vi "remoteControlShooter.vi"() -> ()   [LabVIEW 2019]
uses:
  <vilib>/ReMiSYS/ReMiSYS_myRIO-mini/SubVI/gamepadF710/F710.ctl
  <vilib>/ReMiSYS/ReMiSYS_myRIO-mini/SubVI/gamepadF710/stick.ctl
  <vilib>/ReMiSYS/ReMiSYS_myRIO-mini/SubVI/gamepadF710/gamepadF710.lvclass
  <vilib>/Platform/TimedLoop/XDataNode/timing_clust.ctl
  <vilib>/Platform/TimedLoop/XDataNode/nitl_modes.ctl
  <vilib>/Platform/TimedLoop/XDataNode/wakeup.ctl
  <vilib>/ReMiSYS/ReMiSYS_myRIO-mini/SubVI/SYS/servoPort.ctl
  <vilib>/myRIO/Common/Instrument Driver Framework/myRIO v1.0/UART/vis/myRIO v1.0 Close UART.vi
  <vilib>/myRIO/Common/Instrument Driver Framework/Utilities/vis/FPGA Ref Manager.vi
  <vilib>/myRIO/Common/Instrument Driver Framework/myRIO v1.0/myRIO v1.0 Reset FPGA.vi
  <vilib>/myRIO/Common/Instrument Driver Framework/myRIO v1.0/IRQ/vis/myRIO v1.0 IRQ Info FGV.vi
  <vilib>/myRIO/Common/Instrument Driver Framework/myRIO v1.0/IRQ/vis/myRIO v1.0 Timer IRQ Info FGV.vi
  <vilib>/myRIO/Common/Instrument Driver Framework/myRIO v1.0/IRQ/vis/myRIO v1.0 ISR Agent.vi
  <vilib>/myRIO/Instrument Drivers/Utilities/vis/Reset Index.vi
  <vilib>/myRIO/Common/Instrument Driver Framework/myRIO v1.0/Resource Manager/vis/myRIO v1.0 Block Write Resource Manager.vi
  <vilib>/Platform/TimedLoop/XDataNode/XDataNode.xnode
  <vilib>/Platform/TimedLoop/XDataNode/XDNodeRunTimeDep.lvlib
  <vilib>/myRIO/Instrument Drivers/Utilities/Utilities.lvlib
  <vilib>/vision/Image Controls.llb/IMAQ Image.ctl
panel:
  out "Image Out":T1(plugin-control)
  out "sorted circles by center x then y":T2(array[cluster])
  out "i":i32
  in  "Circle Descriptor (Shape Detection 1)":cluster{"Min Radius":dbl, "Max Radius":dbl}={"Min Radius"=30.0, "Max Radius"=300.0}
  in  "read image\nalgorithm":bool=TRUE
  out "error out":errorcluster
  out "Position.x":sgl
  out "Position.y":sgl
  out "F710 button info.LogiB":bool
  in  "speed 1~10":dbl=10.0
  out "shooterPitch":dbl
  out "ClipCtrl":bool[](array[boolean])
  out "Speed Array":dbl[](array[numeric])
  in  "stop Control?":bool
  out "F710":T3
  out "ENC [L, R, B] (deg)":dbl[](array[numeric])
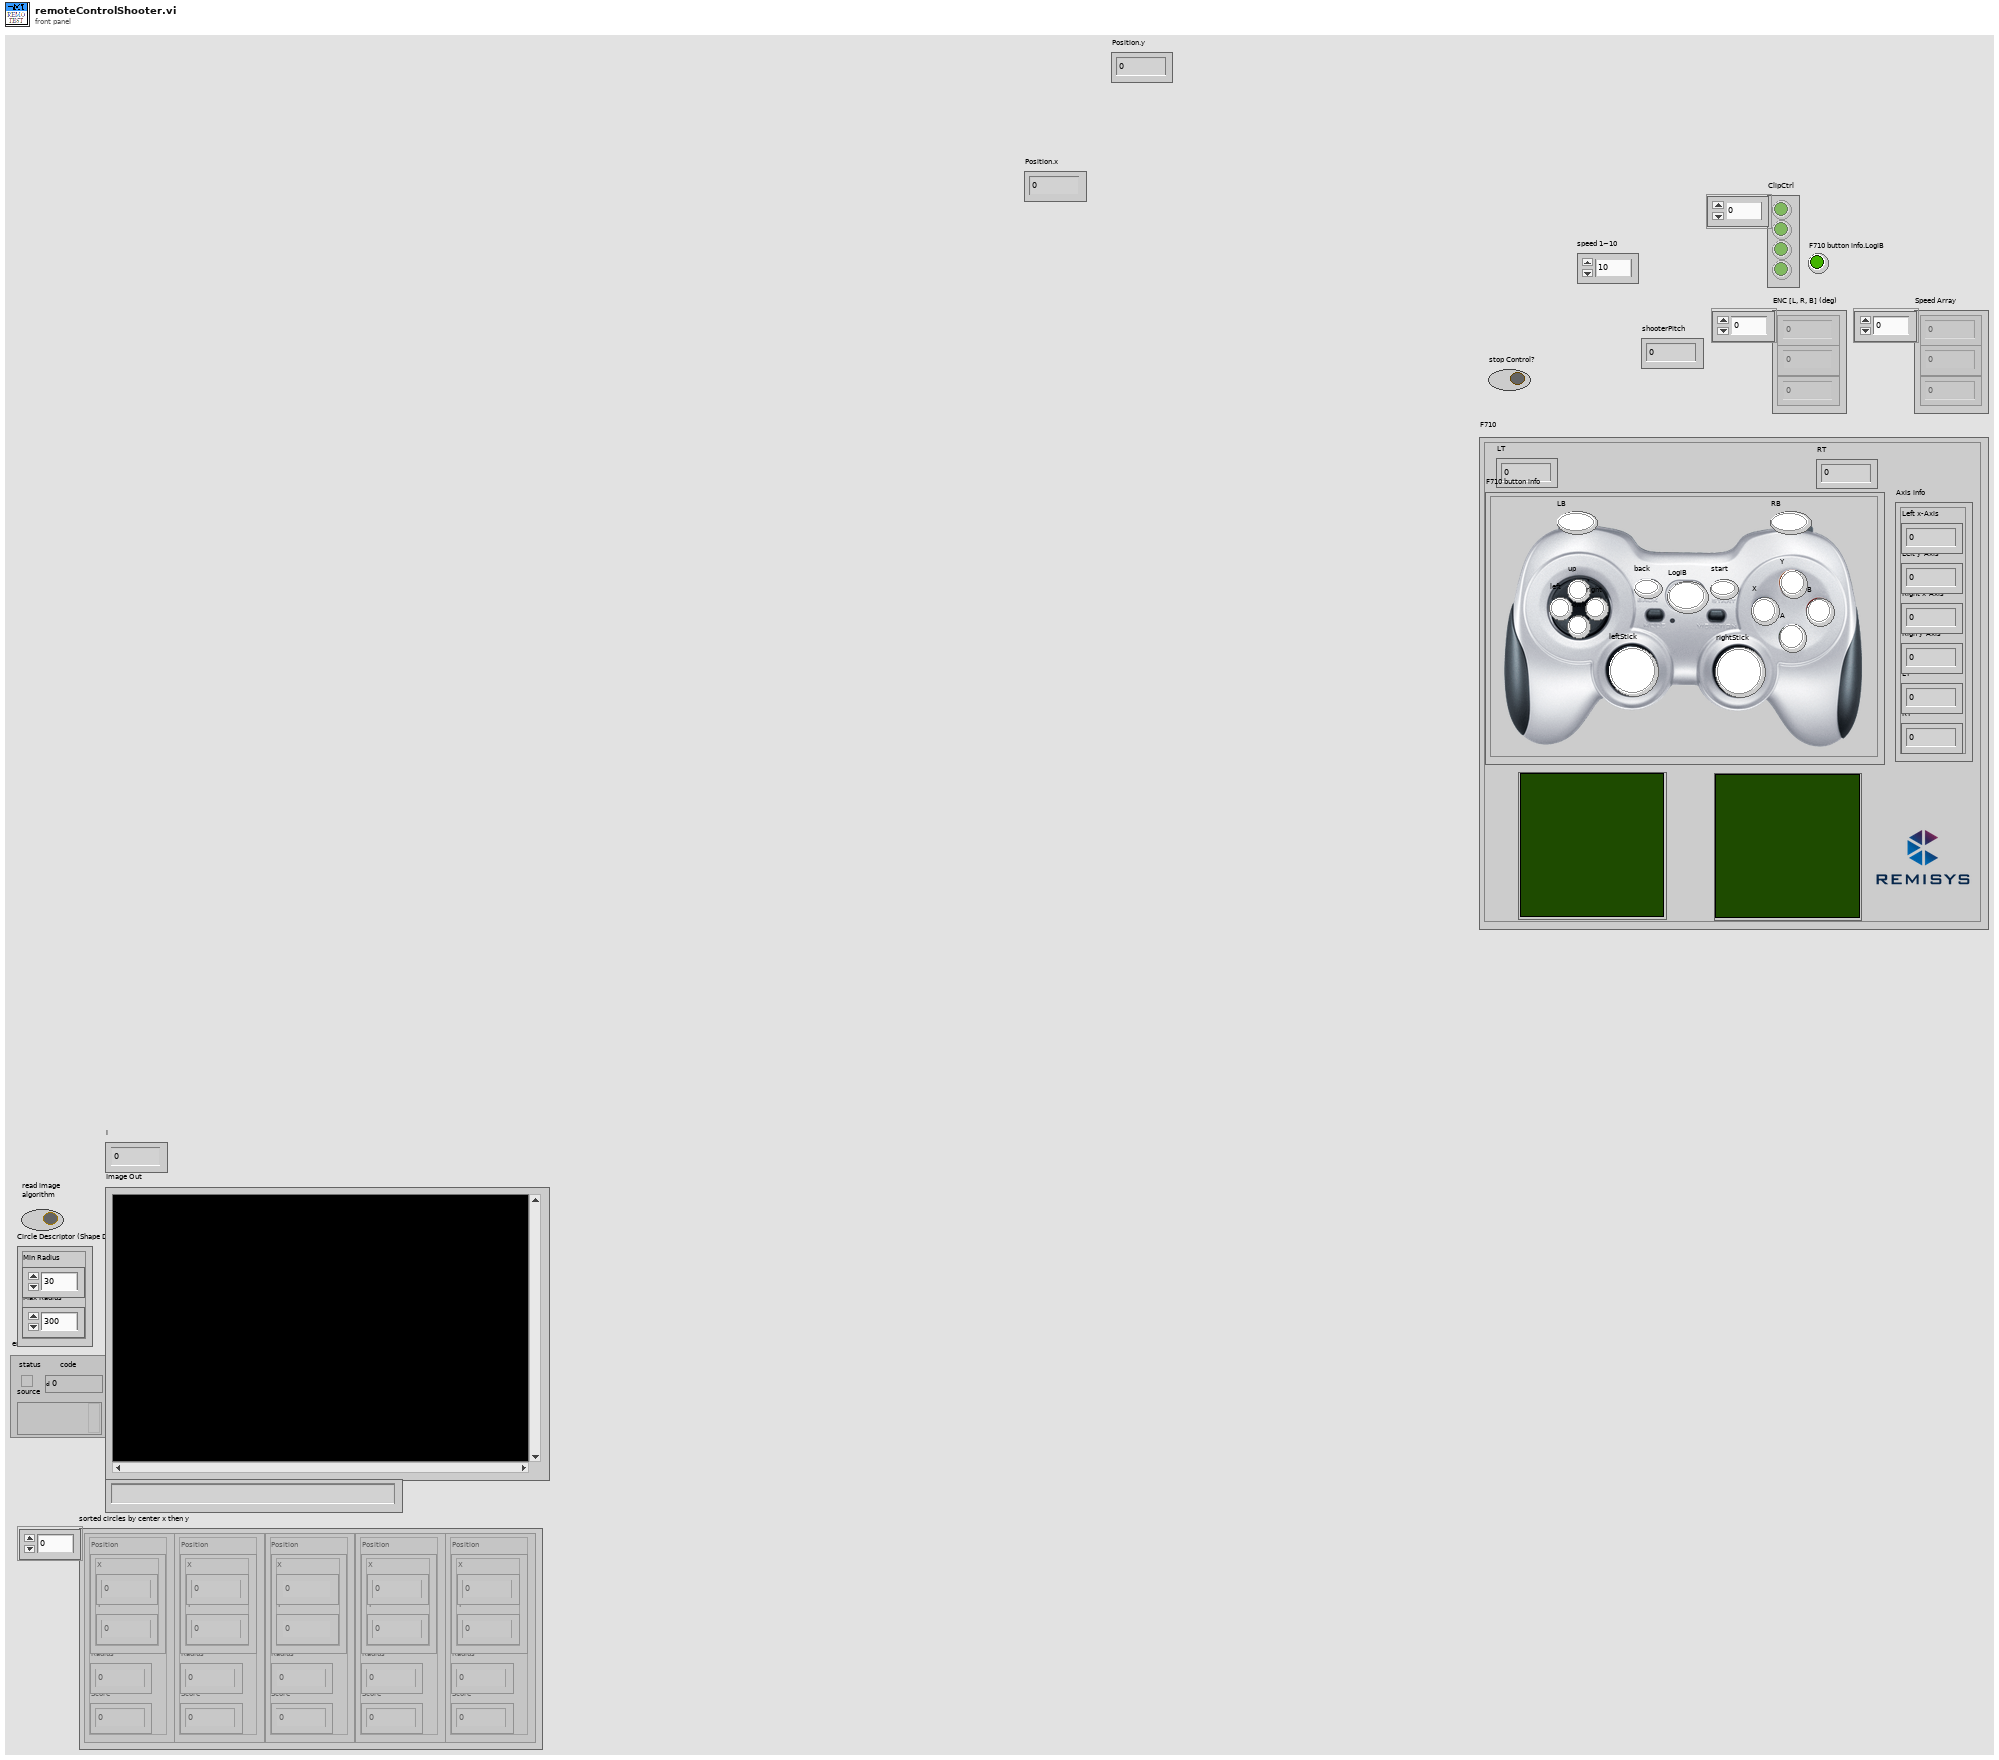
[diagram p1: front panel]
types:
  T1 = typedef "IMAQ Image.ctl" = refnum<image>
  T2 = cluster{"Position":cluster{"X":u16, "Y":u16}, "Radius":u16, "Score":u16}[]
  T3 = typedef "F710.ctl" = cluster{"RT":u8, "LT":u8, "RightStick":T4, "LeftStick":T4, "Axis info":cluster{"Left x-Axis":i8, "Left y-Axis":i8, "Right x-Axis":i8, "Righ y-Axis":i8, "LT":u8, "RT":u8}, "F710 button info":cluster{"RB":bool, "LB":bool, "rightStick":bool, "leftStick":bool, "start":bool, "back":bool, "right":bool, "left":bool, "down":bool, "up":bool, "Y":bool, "X":bool, "B":bool, "A":bool, "LogiB":bool}}
  T4 = typedef "stick.ctl" = cluster{"X":dbl, "Y":dbl}[]
  T5 = cluster{"Position":cluster{"X":sgl, "Y":sgl}, "Radius":dbl, "Score":dbl}[]
  T6 = typedef "Image Type" = u32
  T7 = cluster{"Position":cluster{"X":u16, "Y":u16}, "Radius":u16, "Score":u16}
  T8 = typedef "servoPort.ctl" = enum16{"S1", "S2", "S3", "S4", "S5", "S6", "S7", "S8", "S9"}
  T9 = typedef "XDNodeRunTimeDep.lvlib/timing_clust.ctl" = cluster{"Expected End [f-1]":u64, "Actual End [f-1]":u64, "Finished Late? [f-1]":bool, "Expected End [i-1]":u64, "Actual End [i-1]":u64, "Finished Late? [i-1]":bool, "Expected Start [i]":u64, "Actual Start [i]":u64, "Expected Start [f]":u64, "Actual Start [f]":u64, "Source Name":string, "Structure Name":string, "Period":i64, "Deadline":i64, "Offset":i64, "Start":i64, "Priority":i32, "Timeout":i32, "Mode":T10, "Wakeup Reason":T11, "Error":errorcluster, "Source Type":string, "Secondary Source Type":string, "Global End Time":u64, "Global Start Time":u64, "Frame Duration":u64, "Iteration Duration":u64, "Assigned CPU":i32, "I/O Scan Engine Mode":u32}
  T10 = typedef "XDNodeRunTimeDep.lvlib/nitl_modes.ctl" = enum32{"No Change", "Process missed periods, maintain original phase", "Discard missed periods, maintain original phase", "Process missed periods, ignore original phase", "Discard missed periods, ignore original phase"}
  T11 = typedef "XDNodeRunTimeDep.lvlib/wakeup.ctl" = enum32{"Normal", "Aborted", "Asynchronous wakeup", "Timing source error", "Timed loop error", "Timeout"}
  T12 = typedef "miniRef.ctl" = cluster{"Custom FPGA Reference":refnum<k20>, "error out":errorcluster}
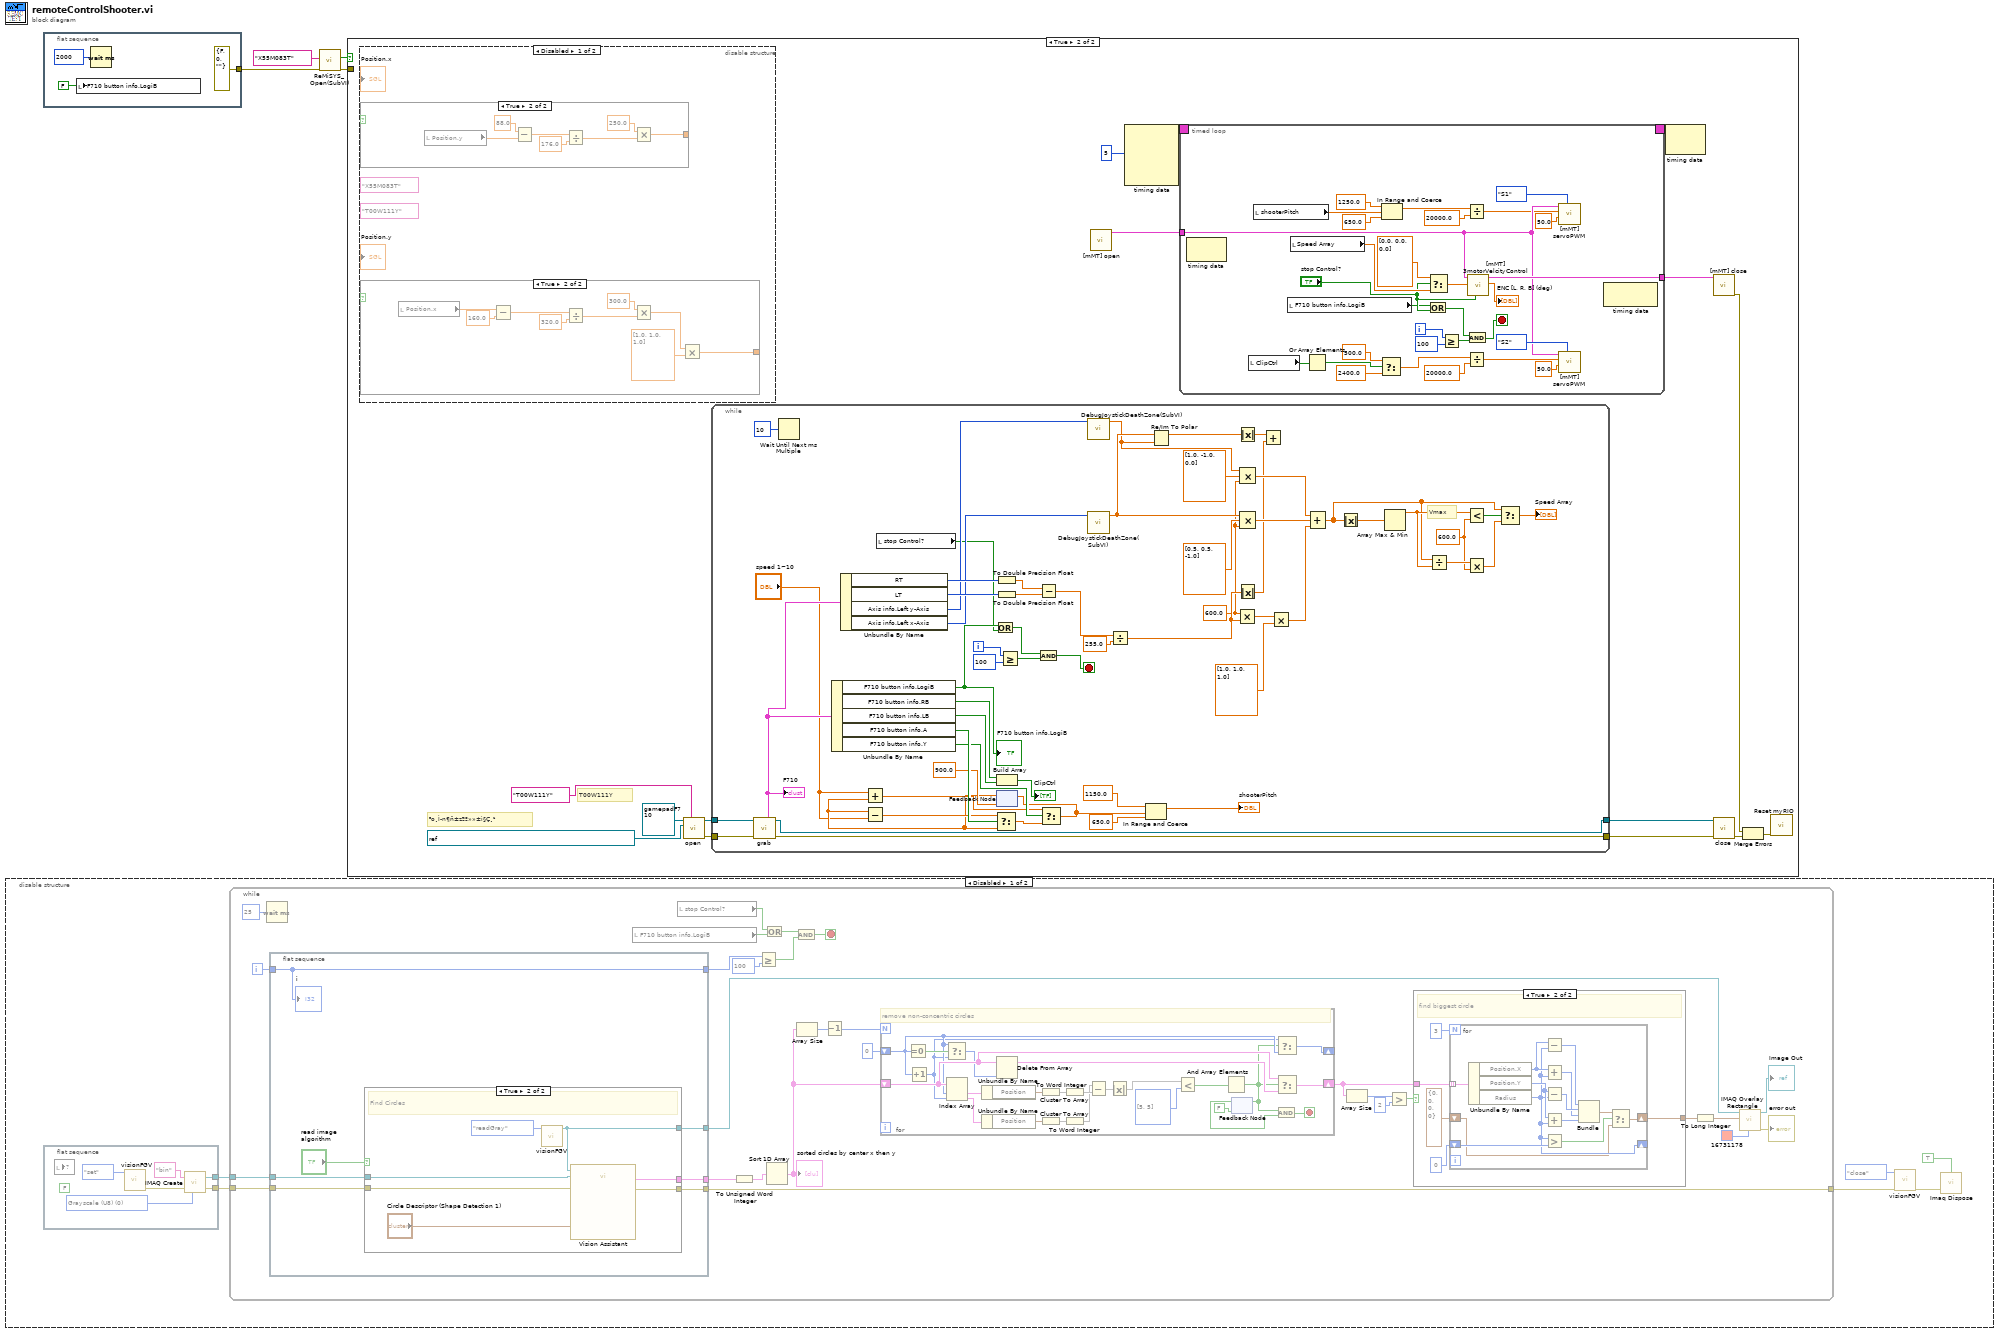
[diagram p0: block diagram]
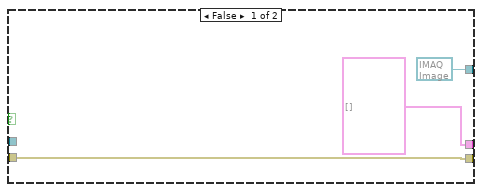
[diagram p2: hidden frame]
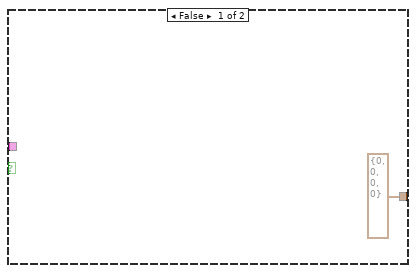
[diagram p3: hidden frame]
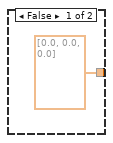
[diagram p6: hidden frame]
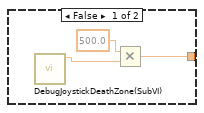
[diagram p7: hidden frame]
diagram:
  n1 = disable-structure shown="Disabled" {
    frame Disabled {
      n2 = flat-sequence {
        tunnel: [w15] -> w10
        tunnel: [w13] -> w7
        frame #0 {
          (unwired) FALSE ("stop Control?")
          w14 = T6 0 items=["Grayscale (U8)", "Grayscale (I16)", "Grayscale (SGL)", "Complex (CSG)", "RGB (U32)", "HSL (U32)", "RGB (U64)", "Grayscale (U16)"] ("Image Type")
          n3 = local read item#-1() -> ()  [unwired: 1 in]
          n4 = call "visionFGV.vi"("Function"=enum16{"set", "readColor", "close", "readGray"}."set") -> ("error out"=w11:errorcluster)  [unwired: 9 in, 1 out]
          n5 = call "IMAQ Create"("Image Name"="bin", "Image Type"=w14, "error in (no error)"=w11) -> ("New Image"=w15:T1, "error out"=w13:errorcluster)  [unwired: 2 in]
        }
      }
      n6 = while {
        tunnel: [w35] -> w6
        tunnel: w10 -> [w44]
        tunnel: w7 -> [w29]
        i -> [w40]
        stop <- w18 stop-if-true
        n7 = Wait (ms)(milliseconds to wait=u32 25) -> ()  [unwired: 1 out]
        n8 = flat-sequence {
          tunnel: [w50] -> w35
          tunnel: [w48] -> w32
          tunnel: [w46] -> w28
          tunnel: w44 -> [w51]
          tunnel: w40 -> [w45]
          tunnel: w29 -> [w47]
          tunnel: [w45] -> w17
          frame #0 {
            n9 = case shown="True" "read image\nalgorithm" {
              tunnel: [w53 w59] -> w50
              tunnel: w51 -> [_ w61]
              tunnel: [T5 [] ("Circles (Shape Detection 1)") w60] -> w48
              tunnel: w47 -> [w53 w57]
              tunnel: [T1 refnum ("Image Out fgv") w55] -> w46
              frame False {
              }
              frame True {
                # "Find Circles"
                n10 = call "visionFGV.vi"("Function"=enum16{"set", "readColor", "close", "readGray"}."readGray") -> ("Image Out fgv"=w55:T1)  [unwired: 9 in, 1 out]
                n11 = call "Vision Assistant"("Image In"=w55, "Image Dst"=w61, "Circle Descriptor (Shape Detection 1)"="Circle Descriptor (Shape Detection 1)", "error in"=w57) -> ("Circles (Shape Detection 1)"=w60:T5, "error out"=w59:errorcluster)  [unwired: 21 in, 1 out]
              }
            }
            "i" <- w45
          }
        }
        n12 = local read "F710 button info.LogiB"() -> (w21:bool)
        n13 = local read "stop Control?"() -> (w22:bool)
        n14 = To Unsigned Word Integer(number=w32) -> (unsigned 16bit integer=w39:T2)
        n15 = Greater Or Equal?(x=w17, y=100) -> (x >= y?=w19:bool)
        n16 = Or(x=w22, y=w21) -> (x .or. y?=w20:bool)
        n17 = Sort 1D Array(array=w39) -> (sorted array=w36:T2)
        "sorted circles by center x then y" <- w36
        n18 = And(x=w20, y=w19) -> (x .and. y?=w18:bool)
        n19 = Array Size(array=w36) -> (size(s)=w38:i32)
        n20 = Decrement(x=w38) -> (x-1=w37:i32)
        n21 = for {
          N: w37 -> [_]
          shift-right: [w81] -> w33
          shift-left: w36 -> [w80]
          shift-right: [w79] -> _
          shift-left: 0 ("index") -> [w76]
          stop <- w70 stop-if-true
          # "remove non-concentric circles"
          n22 = Equal To 0?(x=w76) -> (x = 0?=w77:bool)
          n23 = Increment(x=w76) -> (x+1=w74:i32)
          n24 = Select(t=w76, s=w77, f=w74) -> (s? t:f=w75:i32)
          n25 = Index Array(array=w80, index #1=w76, index #2=w74) -> (element #1=w85:T7, element #2=w83:T7)
          n26 = Unbundle By Name(w85) -> ("Position"=w84:cluster{"X":u16, "Y":u16})
          n27 = Unbundle By Name(w83) -> ("Position"=w82:cluster{"X":u16, "Y":u16})
          n28 = Delete From Array(array=w80, index=w75) -> (array with subset deleted=w78:T2)  [unwired: 1 in, 1 out]
          n29 = Cluster To Array(cluster=w84) -> (array=w68:u16[])
          n30 = Cluster To Array(cluster=w82) -> (array=w69:u16[])
          n31 = To Word Integer(number=w68) -> (16bit integer=w67:i16[])
          n32 = To Word Integer(number=w69) -> (16bit integer=w66:i16[])
          n33 = Subtract(x=w66, y=w67) -> (x-y=w65:i16[])
          n34 = Absolute Value(x=w65) -> (abs(x)=w64:i16[])
          n35 = Less?(x=w64, y=i16[] [5, 5]) -> (x < y?=w62:bool[])
          n36 = And Array Elements(Boolean array=w62) -> (logical AND=w73:bool)
          n37 = feedback-in #1(w73) -> ()
          n38 = feedback #1(FALSE) -> (w72:bool)
          n39 = And(x=w73, y=w72) -> (x .and. y?=w70:bool)
          n40 = Select(t=w74, s=w73, f=w76) -> (s? t:f=w79:i32)
          n41 = Select(t=w80, s=w73, f=w78) -> (s? t:f=w81:T2)
        }
        n42 = Array Size(array=w33) -> (size(s)=w43:i32)
        n43 = Greater?(x=w43, y=2) -> (0:w25:bool)
        n44 = case shown="True" w25 {
          tunnel: w33 -> [_ w89]
          tunnel: [cluster{u16, u16, u16, u16} {0, 0, 0, 0} ("f") w91] -> w30
          frame False {
          }
          frame True {
            # "find biggest circle"
            n45 = for {
              N: 3 ("index") -> [_]
              tunnel: w89 -> [w97] mode=indexing
              shift-right: [w92] -> w91
              shift-left: cluster{u16, u16, u16, u16} {0, 0, 0, 0} -> [w93]
              shift-right: [w94] -> _
              shift-left: u16 0 ("Radius") -> [w95]
              n46 = Unbundle By Name(w97) -> ("Position.X"=w102:u16, "Position.Y"=w100:u16, "Radius"=w94:u16)
              n47 = Subtract(x=w102, y=w94) -> (x-y=w104:u16)
              n48 = Add(x=w102, y=w94) -> (x+y=w101:u16)
              n49 = Subtract(x=w100, y=w94) -> (x-y=w103:u16)
              n50 = Add(x=w100, y=w94) -> (x+y=w99:u16)
              n51 = Greater?(x=w94, y=w95) -> (0:w98:bool)
              n52 = Bundle(w104, w103, w101, w99) -> (w96:cluster{u16, u16, u16, u16})  [unwired: 1 in]
              n53 = Select(t=w96, s=w98, f=w93) -> (s? t:f=w92:cluster{u16, u16, u16, u16})
            }
          }
        }
        n54 = To Long Integer(number=w30) -> (32bit integer=w31:cluster{i32, i32, i32, i32})
        n55 = call "IMAQ Overlay Rectangle"("Color"=u32 16731178, "Rectangle"=w31, "Image"=w28) -> ("error out"=→"error out":errorcluster, "Image Out"=→"Image Out":T1)  [unwired: 7 in]
      }
      n56 = call "visionFGV.vi"("Error In"=w6, "Function"=enum16{"set", "readColor", "close", "readGray"}."close") -> ("error out"=w5:errorcluster)  [unwired: 8 in, 1 out]
      n57 = call "Imaq Dispose"("All Images? (No)"=TRUE, "error in (no error)"=w5) -> ()  [unwired: 4 in, 1 out]
    }
    frame Enabled {
    }
  }
  n58 = flat-sequence {
    tunnel: [errorcluster {"status"=FALSE, "code"=0, "source"=""} ("error in (no error)")] -> w1
    frame #0 {
      n59 = local write "F710 button info.LogiB"(FALSE ("x .or. y?")) -> ()
      n60 = Wait (ms)(milliseconds to wait=u32 2000) -> ()  [unwired: 1 out]
    }
  }
  n61 = call <vilib>:"ReMiSYS_Open(SubVI).vi"("error in (no error)"=w1, "ReMiSYS Key"="X55M083T") -> ("error out"=w4:errorcluster, "Correct Key?"=w3:bool)  [unwired: 8 in]
  n62 = case shown="True" w3 {
    tunnel: w4 -> [_ _]
    frame False {
    }
    frame True {
      # "T00W111Y"
      # "³o¸Ì­n¶ñ±zªº»»±ì§Ç¸¹"
      n63 = disable-structure shown="Disabled" {
        frame Disabled {
          (unwired) "T00W111Y" ("INPUT S/N")
          (unwired) "X55M083T" ("ReMiSYS Key")
          n64 = case shown="True" {
            selector: _ -> [_ _]
            tunnel: [w133 w136] -> _
            frame False {
              n65 = call <vilib>:"DebugJoystickDeathZone(SubVI).vi"() -> ("ValueOut 1~-1"=w135:dbl)  [unwired: 11 in]
              n66 = Multiply(x=500.0, y=w135) -> (x*y=w133:dbl)
            }
            frame True {
              n67 = local read "Position.y"() -> (w140:sgl)
              n68 = Subtract(x=sgl 88.0 ("y"), y=w140) -> (x-y=w139:sgl)
              n69 = Divide(x=w139, y=176.0) -> (x/y=w138:dbl)
              n70 = Multiply(x=250.0 ("pitchSpeed"), y=w138) -> (x*y=w136:dbl)
            }
          }
          n71 = case shown="True" {
            selector: _ -> [_ _]
            tunnel: [dbl[] [0.0, 0.0, 0.0] w129] -> _
            frame False {
            }
            frame True {
              n72 = local read "Position.x"() -> (w132:sgl)
              n73 = Subtract(x=w132, y=sgl 160.0) -> (x-y=w125:sgl)
              n74 = Divide(x=w125, y=320.0) -> (x/y=w124:dbl)
              n75 = Multiply(x=sgl 300.0 ("turnSpeed"), y=w124) -> (x*y=w128:dbl)
              n76 = Multiply(x=w128, y=dbl[] [1.0, 1.0, 1.0]) -> (x*y=w129:dbl[])
            }
          }
        }
        frame Enabled {
        }
      }
      n77 = call <vilib>:"open.vi"("INPUT S/N"="T00W111Y", "VISA resource name"=refnum<visa-resource-name> "USB0::0x046D::0xC21F::A6269818::RAW", "gamepadF710 in"=refnum<class "gamepadF710.lvclass"> refnum) -> ("error out"=w113:errorcluster, "gamepadF710 out"=w117:refnum<class "gamepadF710.lvclass">)  [unwired: 7 in]
      n78 = while {
        tunnel: w117 -> [w200]
        tunnel: [w199] -> w116
        tunnel: w113 -> [w172]
        tunnel: [w171] -> w112
        i -> [w146]
        stop <- w143 stop-if-true
        w166 = 600.0 ("y")
        w162 = 600.0 ("tiltScale")
        # "Vmax"
        n79 = call <vilib>:"grab.vi"("error in (no error)"=w172, "gamepadF710 in"=w200) -> ("error out"=w171:errorcluster, "gamepadF710 out"=w199:refnum<class "gamepadF710.lvclass">, "F710"=w187:T3)  [unwired: 6 in]
        "F710" <- w187
        n80 = Wait Until Next ms Multiple(millisecond multiple=u32 10) -> ()  [unwired: 1 out]
        n81 = Unbundle By Name(w187) -> ("F710 button info.LogiB"=w149:bool, "F710 button info.RB"=w186:bool, "F710 button info.LB"=w185:bool, "F710 button info.A"=w161:bool, "F710 button info.Y"=w160:bool)
        "F710 button info.LogiB" <- w149
        n82 = Unbundle By Name(w187) -> ("RT"=w191:u8, "LT"=w189:u8, "Axis info.Left y-Axis"=w183:i8, "Axis info.Left x-Axis"=w182:i8)
        n83 = local read "stop Control?"() -> (w148:bool)
        n84 = Or(x=w149, y=w148) -> (x .or. y?=w147:bool)
        n85 = To Double Precision Float(number=w191) -> (double precision float=w190:dbl)
        n86 = To Double Precision Float(number=w189) -> (double precision float=w188:dbl)
        n87 = Build Array(w186, w185) -> (→"ClipCtrl":bool[])
        n88 = feedback #2(900.0) -> (w155:dbl)
        n89 = Add(x="speed 1~10", y=w155) -> (x+y=w159:dbl)
        n90 = Subtract(x=w155, y="speed 1~10") -> (x-y=w157:dbl)
        n91 = Select(t=w157, s=w161, f=w155) -> (s? t:f=w158:dbl)
        n92 = Greater Or Equal?(x=w146, y=100) -> (x >= y?=w144:bool)
        n93 = Subtract(x=w190, y=w188) -> (x-y=w181:dbl)
        n94 = And(x=w147, y=w144) -> (x .and. y?=w143:bool)
        n95 = Select(t=w159, s=w160, f=w158) -> (s? t:f=w151:dbl)
        n96 = feedback-in #2(w151) -> ()
        n97 = call <vilib>:"DebugJoystickDeathZone(SubVI).vi"("Axis_Info"=w183) -> ("ValueOut 1~-1"=w178:dbl)  [unwired: 10 in]
        n98 = call <vilib>:"DebugJoystickDeathZone(SubVI).vi"("Axis_Info"=w182) -> ("ValueOut 1~-1"=w179:dbl)  [unwired: 10 in]
        n99 = Divide(x=w181, y=255.0) -> (x/y=w177:dbl)
        n100 = In Range and Coerce(upper limit=1150.0, x=w151, lower limit=650.0) -> (coerced(x)=→"shooterPitch":dbl)  [unwired: 1 out]
        n101 = Re/Im To Polar(2:w178, 3:w179) -> (1:w176:dbl)  [unwired: 1 out]
        n102 = Multiply(x=w162, y=w177) -> (x*y=w163:dbl)
        n103 = Absolute Value(x=w176) -> (abs(x)=w175:dbl)
        n104 = Absolute Value(x=w177) -> (abs(x)=w174:dbl)
        n105 = Compound Arithmetic op=MULTIPLY(w178, dbl[] [1.0, -1.0, 0.0], w162) -> (w194:dbl[])
        n106 = Compound Arithmetic op=MULTIPLY(w179, dbl[] [0.5, 0.5, -1.0], w162) -> (w193:dbl[])
        n107 = Add(x=w175, y=w174) -> ()  [unwired: 1 out]
        n108 = Multiply(x=w163, y=dbl[] [1.0, 1.0, 1.0]) -> (x*y=w192:dbl[])
        n109 = Compound Arithmetic op=ADD(w194, w193, w192) -> (w168:dbl[])
        n110 = Absolute Value(x=w168) -> (abs(x)=w173:dbl[])
        n111 = Array Max & Min(array=w173) -> (max value=w169:dbl)  [unwired: 3 out]
        n112 = Divide(x=w168, y=w169) -> (x/y=w167:dbl[])
        n113 = Less?(x=w169, y=w166) -> (x < y?=w170:bool)
        n114 = Multiply(x=w167, y=w166) -> (x*y=w165:dbl[])
        n115 = Select(t=w168, s=w170, f=w165) -> (s? t:f=→"Speed Array":dbl[])
      }
      n116 = call <vilib>:"[mMT] open.vi"() -> ("miniOut"=w120:T12)  [unwired: 9 in, 2 out]
      n117 = node-c288(i64 5 ("Period")) -> (w122:T9)  [unwired: 3 in]
      n118 = timed-loop {
        tunnel: w120 -> [w221]
        timing: w122 -> [_]
        timing-out: [_] -> w121
        tunnel: [w230] -> w119
        i -> [w203]
        stop <- w201 stop-if-true
        n119 = node-c288() -> ()  [unwired: 1 in, 1 out]
        n120 = local read "ClipCtrl"() -> (w218:bool[])
        n121 = local read "shooterPitch"() -> (w208:dbl)
        n122 = local read "F710 button info.LogiB"() -> (w202:bool)
        n123 = local read "Speed Array"() -> (w228:dbl[])
        n124 = Or Array Elements(Boolean array=w218) -> (logical OR=w217:bool)
        n125 = Select(t=500.0 ("y"), s=w217, f=2400.0 ("y")) -> (s? t:f=w210:dbl)
        n126 = In Range and Coerce(upper limit=1250.0, x=w208, lower limit=650.0) -> (coerced(x)=w213:dbl)  [unwired: 1 out]
        n127 = Or(x=w202, y="stop Control?") -> (x .or. y?=w204:bool)
        n128 = Select(t=dbl[] [0.0, 0.0, 0.0], s="stop Control?", f=w228) -> (s? t:f=w226:dbl[])
        n129 = Greater Or Equal?(x=w203, y=100) -> (x >= y?=w205:bool)
        n130 = Divide(x=w213, y=20000.0) -> (x/y=w214:dbl)
        n131 = Divide(x=w210, y=20000.0) -> (x/y=w209:dbl)
        n132 = And(x=w204, y=w205) -> (x .and. y?=w201:bool)
        n133 = call <vilib>:"[mMT] 3motorVelcityControl.vi"("reset?"="stop Control?", "Speed [L, R, B] (deg/s)"=w226, "miniOut in"=w221) -> ("ENC [L, R, B] (deg)"=→"ENC [L, R, B] (deg)":dbl[], "miniOut out"=w230:T12)  [unwired: 5 in, 2 out]
        n134 = call <vilib>:"[mMT] servoPWM.vi"("servoPort"=servoPort."S1", "Frequency"=50.0, "DutyCycle"=w214, "miniOut in"=w221) -> ()  [unwired: 6 in, 2 out]
        n135 = call <vilib>:"[mMT] servoPWM.vi"("servoPort"=servoPort."S2", "Frequency"=50.0, "DutyCycle"=w209, "miniOut in"=w221) -> ()  [unwired: 6 in, 2 out]
        n136 = node-c288() -> ()  [unwired: 1 in, 1 out]
      }
      n137 = node-c288(w121) -> ()  [unwired: 1 out]
      n138 = call <vilib>:"[mMT] close.vi"("miniOut in"=w119) -> ("error out"=w111:errorcluster)  [unwired: 10 in]
      n139 = call <vilib>:"close.vi"("error in (no error)"=w112, "gamepadF710 in"=w116) -> ("error out"=w110:errorcluster)  [unwired: 8 in, 1 out]
      n140 = Merge Errors(w111, w110) -> (w109:errorcluster)
      n141 = call <vilib>:"Reset myRIO.vi"("error in (no error)"=w109) -> ()  [unwired: 10 in, 1 out]
    }
  }
